vi "sub_cDAQ_main.vi"(8 "error in":errorcluster) -> (0 "error out":errorcluster)   [LabVIEW 2016]
uses:
  ctl/strain_ctl.ctl
  ctl/q_data.ctl
  Global.vi
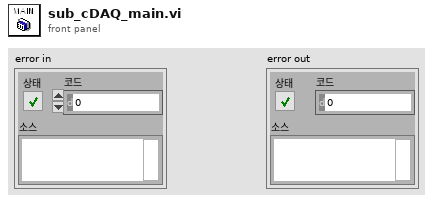
[diagram p1: front panel]
types:
  T1 = typedef "strain_ctl.ctl" = enum16{"config", "start", "read", "close"}
  T2 = typedef "q_data.ctl" = cluster{"Strain raw wf":waveform(dbl)[], "vacuum raw wf":waveform(dbl), "IR raw 2d":i16[][]}
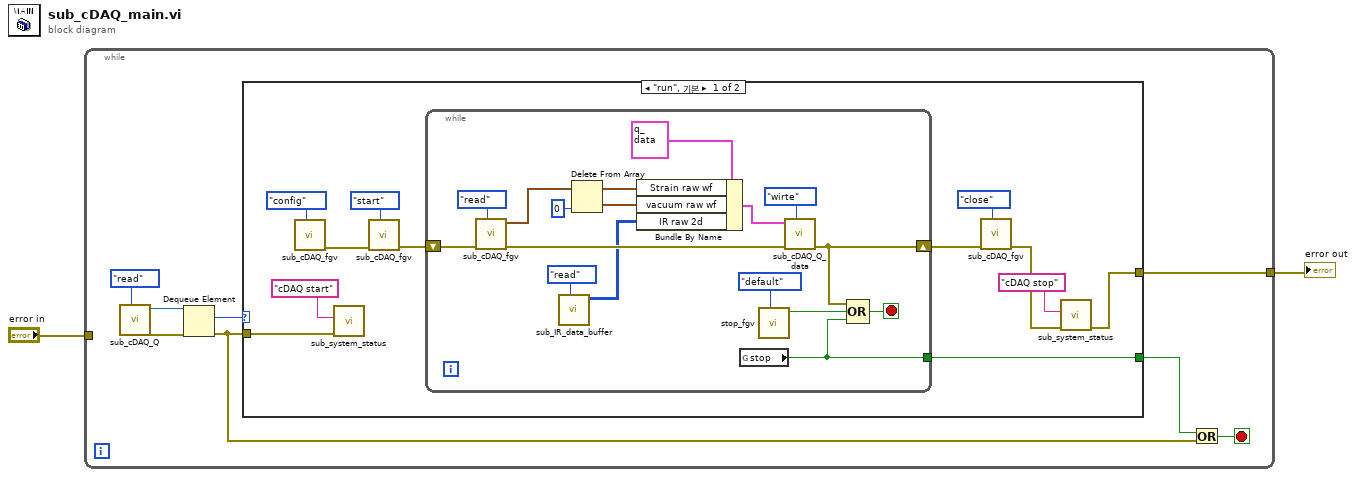
[diagram p0: block diagram]
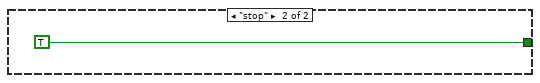
[diagram p2: hidden frame]
diagram:
  n1 = while {
    tunnel: "error in" -> [_]
    tunnel: [w3] -> w2
    stop <- w5 stop-if-true
    n2 = call "sub_cDAQ_Q.vi"("cmd"=enum16{"create", "write", "read", "close"}."read") -> ("error out"=w9:errorcluster, "queue out"=w8:refnum<queue>)  [unwired: 9 in]
    n3 = Dequeue Element(queue=w8, error in (no error)=w9) -> (element=w7:enum16{"run", "stop"}, error out=w4:errorcluster)  [unwired: 1 in, 2 out]
    n4 = case shown="\"run\", 기본" w7 {
      tunnel: [w22 TRUE ("stop")] -> w6
      tunnel: w4 -> [w16 _]
      tunnel: [w11 _] -> w3
      frame "run", Default {
        n5 = call "sub_cDAQ_fgv.vi"("cmd"=strain_ctl."config") -> ("error out"=w19:errorcluster)  [unwired: 9 in, 1 out]
        n6 = call "sub_system_status.vi"("에러 입력(에러 없음)"=w16, "String in"="cDAQ start") -> ()  [unwired: 9 in, 1 out]
        n7 = call "sub_cDAQ_fgv.vi"("cmd"=strain_ctl."start", "error in"=w19) -> ("error out"=w18:errorcluster)  [unwired: 8 in, 1 out]
        n8 = while {
          tunnel: [w34] -> w22
          shift-right: [w31] -> w14
          shift-left: w18 -> [w36]
          stop <- w33 stop-if-true
          n9 = call "sub_cDAQ_fgv.vi"("cmd"=strain_ctl."read", "error in"=w36) -> ("error out"=w32:errorcluster, "data"=w30:waveform(dbl)[])  [unwired: 8 in]
          n10 = call "sub_IR_data_buffer.vi"("cmd"=enum16{"write", "read"}."read") -> ("IR data out"=w23:i16[][])  [unwired: 10 in]
          n11 = Delete From Array(array=w30, index=0 ("인덱스")) -> (deleted portion=w29:waveform(dbl), array with subset deleted=w27:waveform(dbl)[])  [unwired: 1 in]
          n12 = Bundle By Name(cluster=T2 {"Strain raw wf"=[], "vacuum raw wf"={"t0"=timestamp(0 s since 1904-01-01), "dt"=1.0, "Y"=[]}, "IR raw 2d"=[]} ("Q_data"), "Strain raw wf"=w27, "vacuum raw wf"=w29, "IR raw 2d"=w23) -> (w26:T2)
          n13 = global read "Global.vi" "stop"() -> (w34:bool)
          n14 = call "stop_fgv.vi"("cmd"=enum16{"default", "ini", "stop"}."default") -> ("stop"=w38:bool)  [unwired: 9 in, 1 out]
          n15 = call "sub_cDAQ_Q_data.vi"("cmd"=enum16{"create", "wirte", "read", "close"}."wirte", "error in"=w32, "Q_data"=w26) -> ("error out"=w31:errorcluster)  [unwired: 7 in, 1 out]
          n16 = Compound Arithmetic op=OR(w31, w38, w34) -> (w33:bool)
        }
        n17 = call "sub_cDAQ_fgv.vi"("cmd"=strain_ctl."close", "error in"=w14) -> ("error out"=w12:errorcluster)  [unwired: 8 in, 1 out]
        n18 = call "sub_system_status.vi"("에러 입력(에러 없음)"=w12, "String in"="cDAQ stop") -> ("에러 출력"=w11:errorcluster)  [unwired: 9 in]
      }
      frame "stop" {
      }
    }
    n19 = Or(x=w6, y=w4) -> (x .or. y?=w5:bool)
  }
  "error out" <- w2
